vi "Drop.vi"(6 "Copy?":bool, 7 "BetterHandle in (source)":refnum<class "BetterHandle.lvclass">, 8 "error in (no error)":errorcluster, 9 "DragOver Output":T1={"Displayed Row"=0, "Position"=enum."On Row", "Row's TreeItem index"=0, "indent"=0, "Accepted?"=FALSE, "Insertion index"=0, "Top left visible TreeItem index"=0, "Bar type"=enum."tilda up"}, 10 "BetterHandle in (destination)":refnum<class "BetterHandle.lvclass">, 11 "BetterDropOp in":refnum<class "BetterDropOp.lvclass">) -> (0 "error out":errorcluster, 2 "BetterHandle out (destination)":refnum<class "BetterHandle.lvclass">, 3 "BetterDropOp out":refnum<class "BetterDropOp.lvclass">, 5 "BetterHandle out (source)":refnum<class "BetterHandle.lvclass">)   [LabVIEW 2020, in "BetterDragAndDrop.lvlib" / "BetterDropOp.lvclass"]
uses:
  BetterDropOp.lvclass
  SubVIs/DragOver Output.ctl
  SubVIs/DragOverPosition.ctl
  BetterTreeBar/SubVIs/Horizontal Bar Enumeration.ctl
  BetterHandle/BetterHandle.lvclass
  BetterTreeBar/BetterHorizontalBar.lvclass
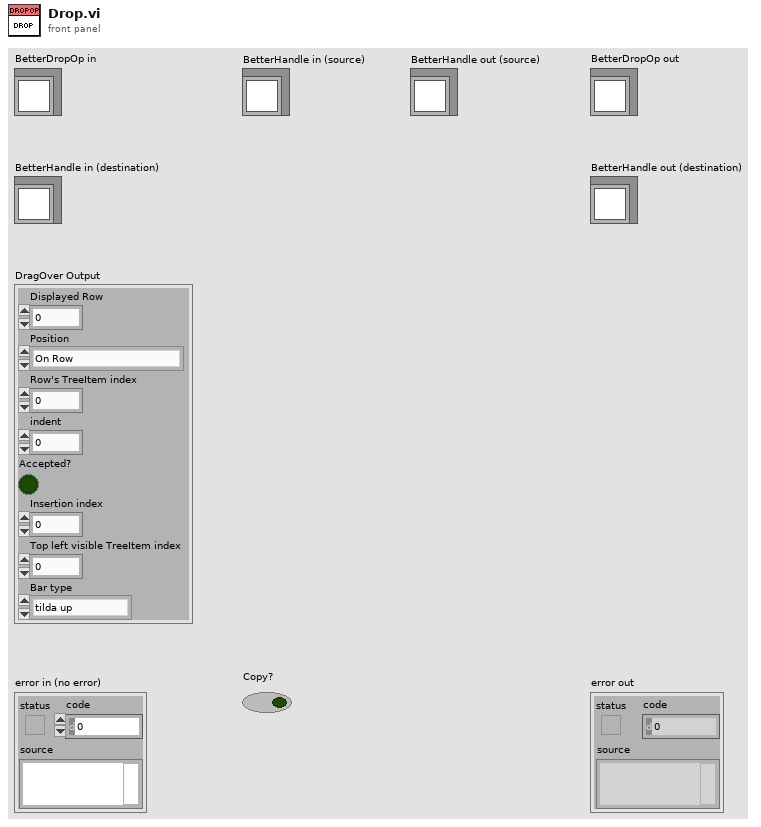
[diagram p1: front panel]
types:
  T1 = typedef "BetterDragAndDrop.lvlib/BetterHandle.lvclass/DragOver Output.ctl" = cluster{"Displayed Row":i32, "Position":T2, "Row's TreeItem index":i32, "indent":i32, "Accepted?":bool, "Insertion index":i32, "Top left visible TreeItem index":i32, "Bar type":T3}
  T2 = typedef "BetterDragAndDrop.lvlib/BetterHandle.lvclass/DragOverPosition.ctl" = enum16{"On Row", "Inbetween"}
  T3 = typedef "BetterDragAndDrop.lvlib/BetterHorizontalBar.lvclass/Horizontal Bar Enumeration.ctl" = enum16{"None", "only bar", "tilda up"}
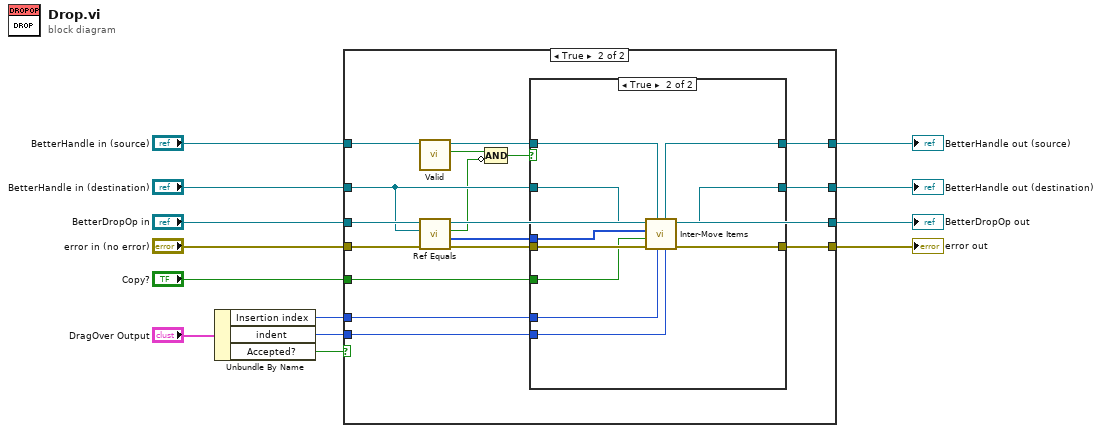
[diagram p0: block diagram]
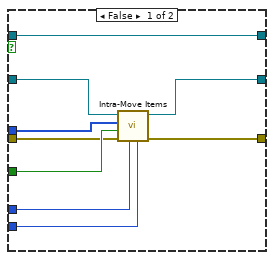
[diagram p3: hidden frame]
diagram:
  n1 = Unbundle By Name("DragOver Output") -> ("Insertion index"=w11:i32, "indent"=w12:i32, "Accepted?"=w13:bool)
  n2 = case shown="True" w13 {
    tunnel: [w16 w34] -> w8
    tunnel: [w17 w33] -> w3
    tunnel: w12 -> [_ w32]
    tunnel: w11 -> [_ w31]
    tunnel: "BetterDropOp in" -> [w14 w30]
    tunnel: "BetterHandle in (destination)" -> [w17 w29]
    tunnel: "Copy?" -> [_ w27]
    tunnel: "error in (no error)" -> [w16 w26]
    tunnel: "BetterHandle in (source)" -> [w15 w22]
    tunnel: [w15 w24] -> w2
    tunnel: [w14 w23] -> w5
    frame False {
    }
    frame True {
      n3 = call "Valid.vi"("BetterHandle In"=w22) -> ("Valid handle?"=w20:bool, "BetterHandle Out"=w21:refnum<class "BetterHandle.lvclass">)  [unwired: 8 in, 1 out]
      n4 = call "Ref Equals.vi"("error in (no error)"=w26, "BetterHandle in"=w29, "BetterDropOp in"=w30) -> ("error out"=w25:errorcluster, "DragStart Indices"=w28:i32[], "Ref is same?"=w19:bool, "BetterDropOp out"=w23:refnum<class "BetterDropOp.lvclass">)  [unwired: 5 in]
      n5 = Compound Arithmetic op=AND(w20, invert w19) -> (w18:bool)
      n6 = case shown="True" w18 {
        tunnel: [w37 w53] -> w34
        tunnel: [w38 w49] -> w33
        tunnel: w32 -> [w40 w44]
        tunnel: w31 -> [w41 w45]
        tunnel: w29 -> [w43 w48]
        tunnel: w28 -> [w39 w47]
        tunnel: w27 -> [w42 w46]
        tunnel: w25 -> [w36 w52]
        tunnel: w21 -> [w35 w51]
        tunnel: [w35 w50] -> w24
        frame False {
          n7 = call-dynamic "Intra-Move Items.vi"("indent"=w40, "Insertion index"=w41, "error in (no error)"=w36, "Copy?"=w42, "Indices to move"=w39, "BetterHandle in"=w43) -> ("error out"=w37:errorcluster, "BetterHandle out"=w38:refnum<class "BetterHandle.lvclass">)  [unwired: 4 in]
        }
        frame True {
          n8 = call "Inter-Move Items.vi"("indent"=w44, "Insertion index"=w45, "BetterHandle in (source)"=w51, "error in (no error)"=w52, "Copy?"=w46, "Indices to move"=w47, "BetterHandle in (destination)"=w48) -> ("error out"=w53:errorcluster, "BetterHandle out (destination)"=w49:refnum<class "BetterHandle.lvclass">, "BetterHandle out (source)"=w50:refnum<class "BetterHandle.lvclass">)  [unwired: 2 in]
        }
      }
    }
  }
  "error out" <- w8
  "BetterDropOp out" <- w5
  "BetterHandle out (destination)" <- w3
  "BetterHandle out (source)" <- w2
